vi "Set Waveform Graph Plot Properties.vi"(10 "Refnums for FP Objects":T4, 11 "State in":T1 caption="State") -> (3 "State out":T1 caption="State")   [LabVIEW 2017, in "Waveforms with Cursors.xctl"]
uses:
  <vilib>/addons/_XControls/Waveforms with Cursors/Waveforms with Cursors.xctl
  <vilib>/addons/_XControls/Waveforms with Cursors/Controls/Refnums Typedef.ctl
  <vilib>/addons/_XControls/Waveforms with Cursors/Controls/State.ctl
  <vilib>/Utility/miscctls.llb/LVFontTypeDef.ctl
  <vilib>/addons/_XControls/Waveforms with Cursors/Controls/Waveform Cursor Configuration.ctl
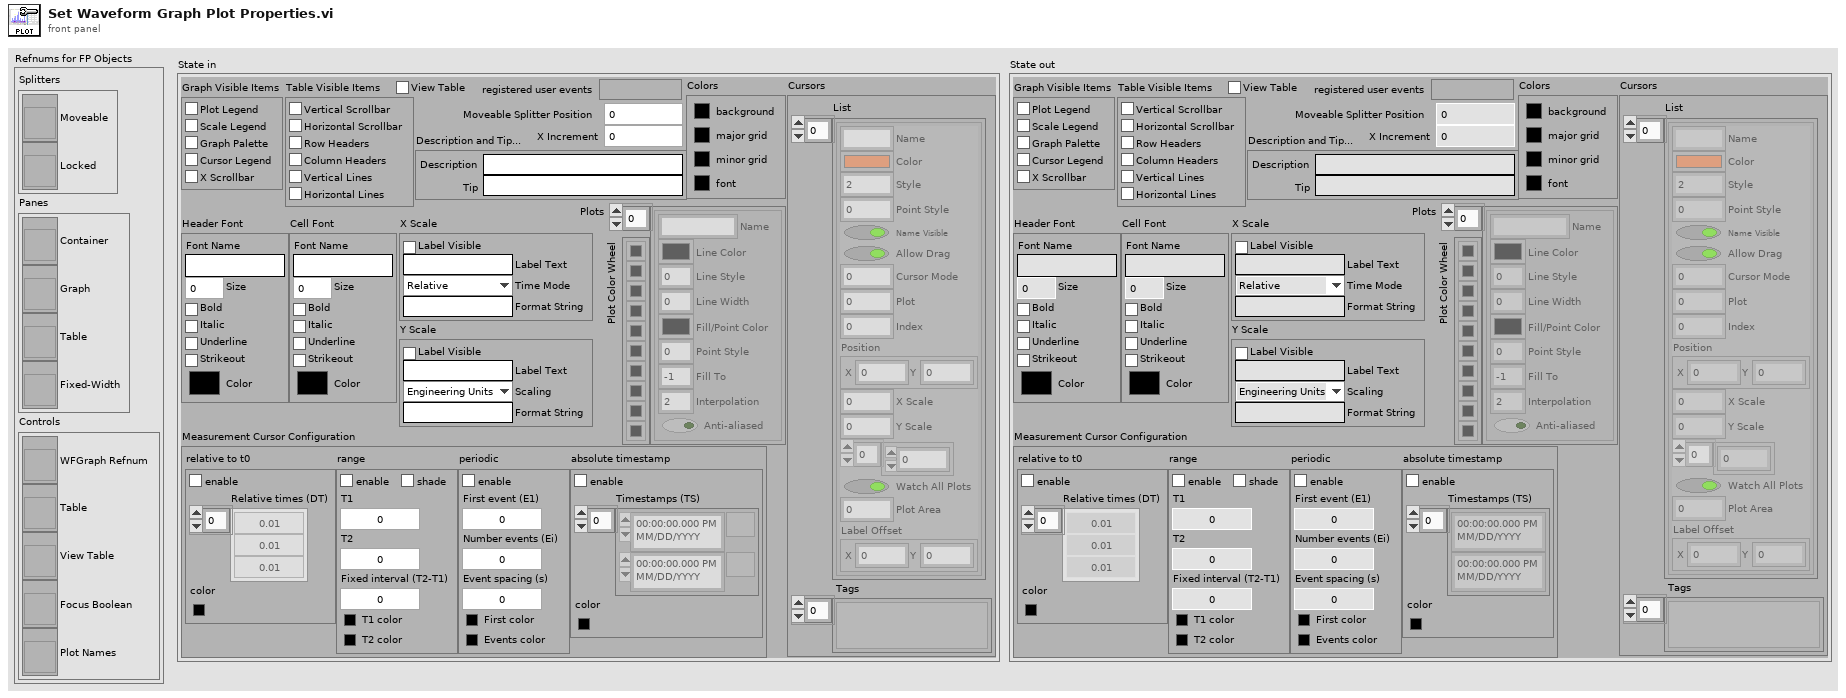
[diagram p1: front panel]
types:
  T1 = typedef "Waveforms with Cursors.xctl/State.ctl" = cluster{"Graph Visible Items":cluster{"Plot Legend":bool, "Scale Legend":bool, "Graph Palette":bool, "Cursor Legend":bool, "X Scrollbar":bool}, "View Table":bool, "Table Visible Items":cluster{"Vertical Scrollbar":bool, "Horizontal Scrollbar":bool, "Row Headers":bool, "Column Headers":bool, "Vertical Lines":bool, "Horizontal Lines":bool}, "Header Font":T2, "Cell Font":T2, "Description and Tip...":cluster{"Description":string, "Tip":string}, "Moveable Splitter Position":i32, "Measurement Cursor Configuration":T3, "X Increment":dbl, "X Scale":cluster{"Label Visible":bool, "Label Text":string, "Time Mode":enum16{"Relative", "Absolute"}, "Format String":string}, "Y Scale":cluster{"Label Visible":bool, "Label Text":string, "Scaling":enum16{"Engineering Units", "Voltage"}, "Format String":string}, "Colors":cluster{"background":u32, "major grid":u32, "minor grid":u32, "font":u32}, "Cursors":cluster{"List":cluster{"Name":string, "Color":u32, "Style":i32, "Point Style":u8, "Name Visible":bool, "Allow Drag":bool, "Cursor Mode":u32, "Plot":i32, "Index":i32, "Position":cluster{"X":dbl, "Y":dbl}, "X Scale":u32, "Y Scale":u32, "Watch Plots":i32[], "Watch All Plots":bool, "Plot Area":i32, "Label Offset":cluster{"X":dbl, "Y":dbl}}[], "Tags":variant[]}, "Plots":cluster{"Name":string, "Line Color":u32, "Line Style":u8, "Line Width":u8, "Fill/Point Color":u32, "Point Style":u8, "Fill To":i16, "Interpolation":u8, "Anti-aliased":bool}[], "Plot Color Wheel":u32[], "registered user events":variant}
  T2 = typedef "LVFontTypeDef.ctl" = cluster{"Font Name":string, "Size":u16, "Bold":bool, "Italic":bool, "Underline":bool, "Strikeout":bool, "Color":u32}
  T3 = typedef "Waveforms with Cursors.xctl/Waveform Cursor Configuration.ctl" = cluster{"relative to t0":cluster{"enable relative time":bool, "Relative times (DT)":dbl[], "color":u32}, "range":cluster{"enable range":bool, "T1":dbl, "T2":dbl, "Fixed interval (T2-T1)":dbl, "T1 color":u32, "T2 color":u32, "enable shading":bool}, "periodic":cluster{"enable periodic":bool, "First event (E1)":dbl, "Number events (Ei)":i32, "Event spacing (s)":dbl, "First color":u32, "Events color":u32}, "absolute timestamp":cluster{"enable absolute":bool, "Timestamps (TS)":timestamp[], "color":u32}}
  T4 = typedef "Waveforms with Cursors.xctl/Refnums Typedef.ctl" = cluster{"Splitters":cluster{"Moveable":refnum<vi>, "Locked":refnum<vi>}, "Panes":cluster{"Container":refnum<vi>, "Graph":refnum<vi>, "Table":refnum<vi>, "Fixed-Width":refnum<vi>}, "Controls":cluster{"WFGraph Refnum":refnum<vi>, "Table":refnum<vi>, "View Table":refnum<vi>, "Focus Boolean":refnum<vi>, "Plot Names":refnum<vi>}}
  T5 = cluster{"Name":string, "Line Color":u32, "Line Style":u8, "Line Width":u8, "Fill/Point Color":u32, "Point Style":u8, "Fill To":i16, "Interpolation":u8, "Anti-aliased":bool}[]
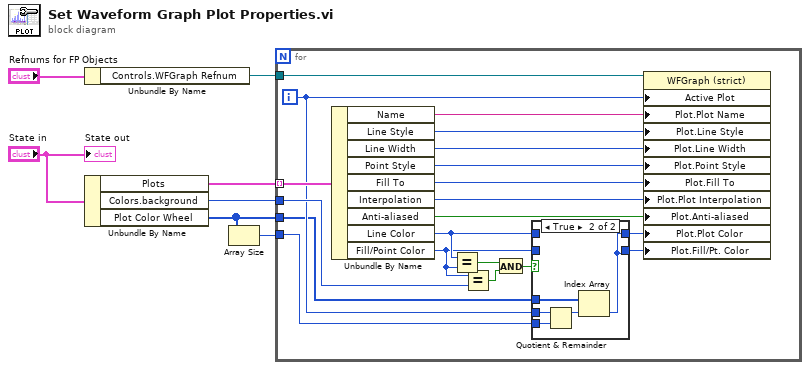
[diagram p0: block diagram]
diagram:
  n1 = Unbundle By Name("Refnums for FP Objects") -> ("Controls.WFGraph Refnum"=w2:refnum<vi>)
  n2 = Unbundle By Name("State in") -> ("Plots"=w3:T5, "Colors.background"=w5:u32, "Plot Color Wheel"=w6:u32[])
  n3 = Array Size(array=w6) -> (size(s)=w7:i32)
  n4 = for {
    tunnel: w2 -> [w27]
    tunnel: w3 -> [w26] mode=indexing
    tunnel: w6 -> [w13]
    tunnel: w5 -> [w18]
    tunnel: w7 -> [w12]
    i -> [w15]
    n5 = Unbundle By Name(w26) -> ("Name"=w25:string, "Line Style"=w24:u8, "Line Width"=w23:u8, "Point Style"=w22:u8, "Fill To"=w21:i16, "Interpolation"=w20:u8, "Anti-aliased"=w19:bool, "Line Color"=w11:u32, "Fill/Point Color"=w9:u32)
    n6 = Equal?(x=w11, y=w9) -> (x = y?=w17:bool)
    n7 = Equal?(x=w9, y=w18) -> (x = y?=w16:bool)
    n8 = And(x=w17, y=w16) -> (x .and. y?=w14:bool)
    n9 = case shown="True" w14 {
      tunnel: w15 -> [_ w33]
      tunnel: w13 -> [_ w32]
      tunnel: w12 -> [_ w31]
      tunnel: w11 -> [w28 _]
      tunnel: [w28 w30] -> w10
      tunnel: w9 -> [w29 _]
      tunnel: [w29 w30] -> w8
      frame False {
      }
      frame True {
        n10 = Quotient & Remainder(x=w33, y=w31) -> (x-y*floor(x/y)=w34:i32)  [unwired: 1 out]
        n11 = Index Array(array=w32, index=w34) -> (element=w30:u32)
      }
    }
    n12 = property class="WFGraph (strict)"(reference=w27, "Active Plot"=w15, "Plot.Plot Name"=w25, "Plot.Line Style"=w24, "Plot.Line Width"=w23, "Plot.Point Style"=w22, "Plot.Fill To"=w21, "Plot.Plot Interpolation"=w20, "Plot.Anti-aliased"=w19, "Plot.Plot Color"=w10, "Plot.Fill/Pt. Color"=w8) -> ()  [unwired: 1 in, 2 out]
  }
  "State out" <- "State in"
